vi "niRFUtil MEAS Max and Min (real wfm).vi"(2 "Waveform In":T1 {"y" min=0 max=127 format="%.2f"; "dx" format="%^.2e"; "x0" format="%^.2e"}) -> (6 "Max":sgl format="%.2f", 7 "Min":sgl format="%.2f")   [LabVIEW 2015, in "niRFUtil.lvlib"]
doc: "(c) Copyright 2006, National Instruments, Inc. This VI may not be duplicated, sold, or distributed without written consent from National Instruments."
uses:
  niRFUtil.lvlib
  Includes/niRFUtil INC Real Waveform.ctl
  Includes/niRFUtil INC Real Array.ctl
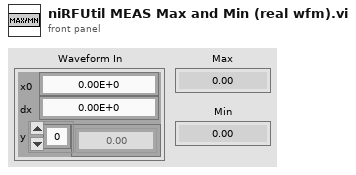
[diagram p1: front panel]
types:
  T1 = typedef "niRFUtil.lvlib/niRFUtil INC Real Waveform.ctl" = cluster{"x0":dbl, "dx":dbl, "y":T2}
  T2 = typedef "niRFUtil.lvlib/niRFUtil INC Real Array.ctl" = sgl[]
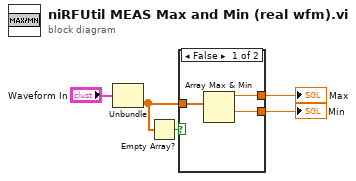
[diagram p0: block diagram]
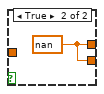
[diagram p2: hidden frame]
diagram:
  n1 = Unbundle("Waveform In") -> ("y"=w2:T2)  [unwired: 2 out]
  n2 = Empty Array?(array=w2) -> (empty?=w1:bool)
  n3 = case shown="False" w1 {
    tunnel: w2 -> [w8 _]
    tunnel: [w7 w9] -> w4
    tunnel: [w6 w9] -> w3
    frame False {
      n4 = Array Max & Min(array=w8) -> (max value=w7:sgl, min value=w6:sgl)  [unwired: 2 out]
    }
    frame True {
      w9 = sgl nan
    }
  }
  "Max" <- w4
  "Min" <- w3
